vi "Algorithm Result User Event_RC.vi"(8 "error in (no error)":errorcluster, 10 "Algorithm Result Data":T1, 11 "Rack Controller in":refnum<class "Rack Controller.lvclass">) -> (0 "error out":errorcluster, 3 "Rack Controller out":refnum<class "Rack Controller.lvclass">)   [LabVIEW 2019, in "Rack Controller.lvclass"]
uses:
  Rack Controller.lvclass
  <vilib>/vision/Image Controls.llb/IMAQ Image.ctl
  Controls/Result Cluster_RC.ctl
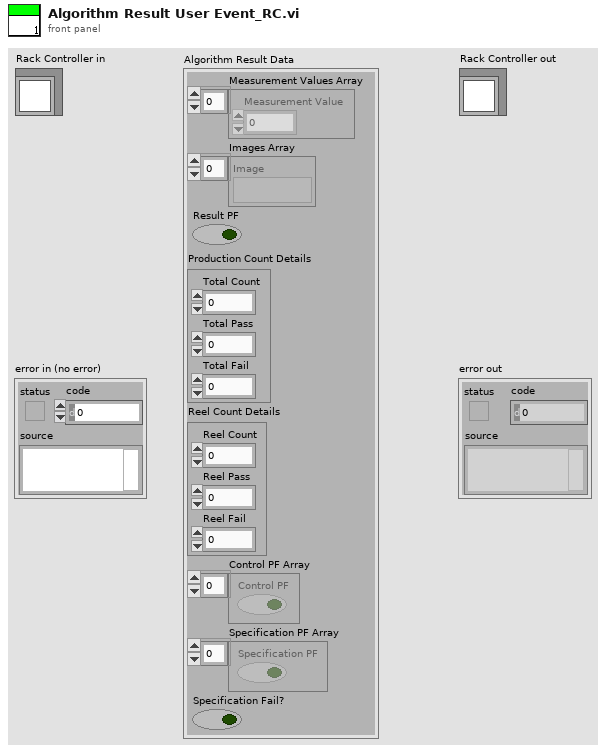
[diagram p1: front panel]
types:
  T1 = typedef "Rack Controller.lvclass/Result Cluster_RC.ctl" = cluster{"Measurement Values Array ":dbl[], "Images Array":T2[], "Result PF":bool, "Production Count Details":cluster{"Total Fail":u64, "Total Pass":u64, "Total Count":u64}, "Reel Count Details":cluster{"Reel Fail":u64, "Reel Pass":u64, "Reel Count":u64}, "Control PF Array":bool[], "Specification PF Array":bool[], "Specification Fail?":bool}
  T2 = typedef "IMAQ Image.ctl" = refnum<image>
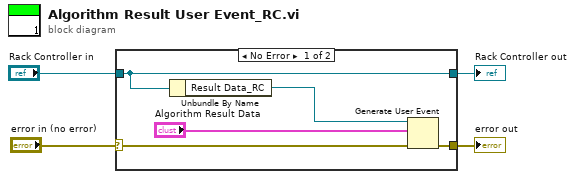
[diagram p0: block diagram]
diagram:
  n1 = case shown="No Error" "error in (no error)" {
    selector: "error in (no error)" -> [w7 w11]
    tunnel: [w6 w11] -> w3
    tunnel: [w9 w10] -> w1
    tunnel: "Rack Controller in" -> [w9 w10]
    frame No Error {
      n2 = Unbundle By Name(w9) -> ("Result Data_RC"=w8:refnum<user-event>)
      n3 = Generate User Event(user event=w8, event data cluster="Algorithm Result Data", error in=w7) -> (error out=w6:errorcluster)  [unwired: 1 in, 1 out]
    }
    frame Error {
    }
  }
  "error out" <- w3
  "Rack Controller out" <- w1
